vi "DataWriteBinGen.vi"(0 "DataFileName":path, 1 "offset (en octets) (0)":i64, 5 "LastScanPosIn":dbl[](array[numeric]), 7 "XY Graph":T1(array[cluster]), 9 "AllYDataIn":dbl[][](array[numeric]), 11 "error in (no error)":errorcluster) -> (8 "XY Graph Out":T1(array[cluster]), 10 "AllYDataOut":dbl[][](array[numeric]), 15 "error out":errorcluster)   [LabVIEW 2010]
doc: "Ce VI sauvegarde les données d'acquisition pour en garder une copie de sécurité qui peut être rappeller en cas de panne."
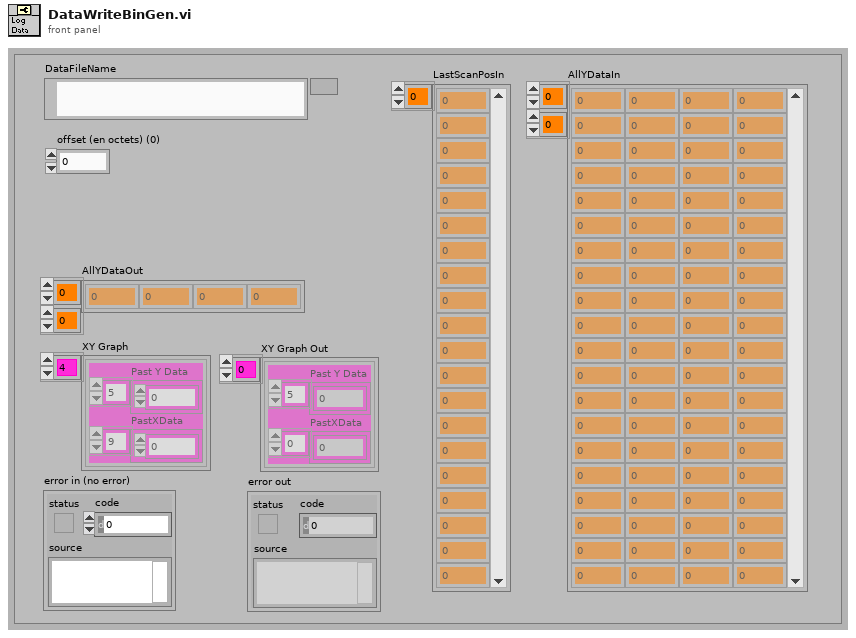
[diagram p1: front panel]
types:
  T1 = cluster{"Past Y Data":dbl[], "PastXData":dbl[]}[]
  T2 = cluster{"AllYDataIn":dbl[][], "XY Graph":cluster{"Past Y Data":dbl[], "PastXData":dbl[]}[], "LastScanPosIn":dbl[]}
  T3 = enum16{"open", "replace", "create", "open or create", "replace or create", "replace or create with confirmation"}
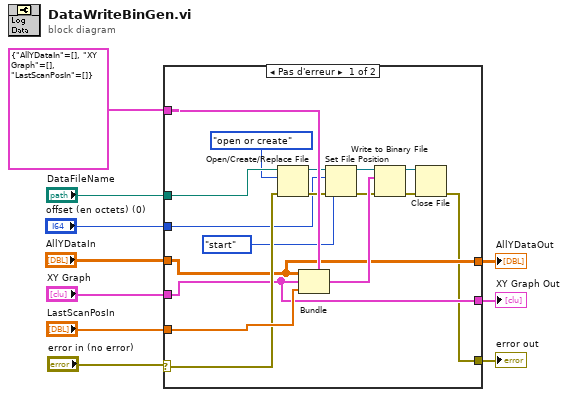
[diagram p0: block diagram]
diagram:
  n1 = case shown="Pas d'erreur" "error in (no error)" {
    selector: "error in (no error)" -> [w24 w30]
    tunnel: "LastScanPosIn" -> [w25 _]
    tunnel: "AllYDataIn" -> [w16 w29]
    tunnel: "XY Graph" -> [w15 w28]
    tunnel: [w12 w30] -> w6
    tunnel: [w15 w28] -> w5
    tunnel: [w16 w29] -> w4
    tunnel: "DataFileName" -> [w27 _]
    tunnel: T2 {"AllYDataIn"=[], "XY Graph"=[], "LastScanPosIn"=[]} -> [w23 _]
    tunnel: "offset (en octets) (0)" -> [w11 _]
    frame No Error {
      n2 = Open/Create/Replace File(file path (use dialog)=w27, error in=w24, operation (0:open)=T3."open or create" ("opération (0 : open)")) -> (refnum out=w19:refnum<file>, error out=w18:errorcluster)  [unwired: 3 in, 1 out]
      n3 = Bundle(cluster=w23, "AllYDataIn"=w16, "XY Graph"=w15, "LastScanPosIn"=w25) -> (w22:T2)
      n4 = Set File Position(offset (in bytes) (0)=w11, refnum=w19, from (0:start)=enum16{"start", "end", "current"}."start" ("à partir de (0 : start)"), error in=w18) -> (refnum out=w20:refnum<file>, error out=w21:errorcluster)
      n5 = Write to Binary File(file (use dialog)=w20, data=w22, error in=w21) -> (refnum out=w14:refnum<file>, error out=w13:errorcluster)  [unwired: 3 in, 1 out]
      n6 = Close File(refnum=w14, error in=w13) -> (error out=w12:errorcluster)  [unwired: 1 out]
    }
    frame Error {
    }
  }
  "AllYDataOut" <- w4
  "XY Graph Out" <- w5
  "error out" <- w6
